vi "3d_display3.vi"() -> ()   [LabVIEW 2009]
doc: "This example demonstrates some fundamental concepts for the 3D picture control. Concepts covered include:\n\n-Object creation\n-Texturing\n-Object movement\n-Object hierarchy"
uses:
  <vilib>/Utility/miscctls.llb/LVRectTypeDef.ctl
  <vilib>/picture/3D Picture Control/NI_3D Picture Control.lvlib
  <vilib>/Analysis/NI_AALBase.lvlib
panel:
  out "xadd":dbl
  out "zadd":dbl
  out "raw pitot":dbl
  in  "Calibrate pitot":bool
  in  "voltage offset":dbl=2.5
  in  "velocity scale":dbl=10000.0
  in  "Set Start Time (s)":dbl
  in  "X":dbl
  in  "Z":dbl
  in  "Calibrate Z":bool
  in  "Calibrate Y":bool
  in  "Calibrate X":bool
  out "angle 2":dbl
  out "angle 1":dbl
  out "X mean acceleration":dbl format="%0.4f"
  out "Y mean acceleration":dbl format="%0.4f"
  out "X mean volts":dbl format="%0.4f"
  out "Y mean volts":dbl format="%0.4f"
  out "Z mean acceleration":dbl format="%0.4f"
  out "Z mean volts":dbl format="%0.4f"
  in  "z gain":dbl=5.0
  in  "z offset":dbl=1.25
  in  "y gain":dbl=5.0
  in  "y offset":dbl=1.25
  in  "x gain":dbl=5.0
  in  "x offset":dbl=1.25
  in  "Render Dest":enum16{"Scene Window", "Scene Display"}(ring)=enum."Scene Display"
  in  "Camera Controller":enum16{"None", "Spherical", "Flying"}(ring)=enum."Spherical"
  out "Scene Display":refnum<vi>(3d-picture)
  in  "stop":bool
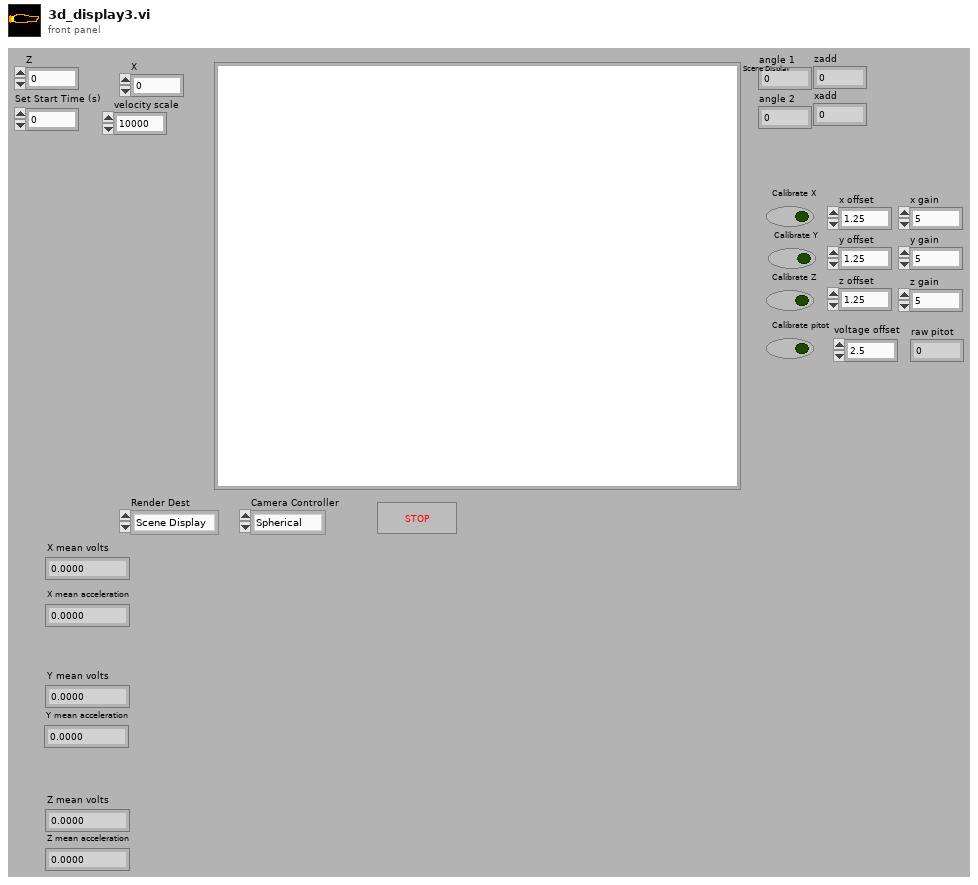
[diagram p1: front panel]
types:
  T1 = typedef "LVRectTypeDef.ctl" = cluster{"Left":i16, "Top":i16, "Right":i16, "Bottom":i16}
  T2 = enum16{"Open", "Minimized", "Maximized", "Hidden"}
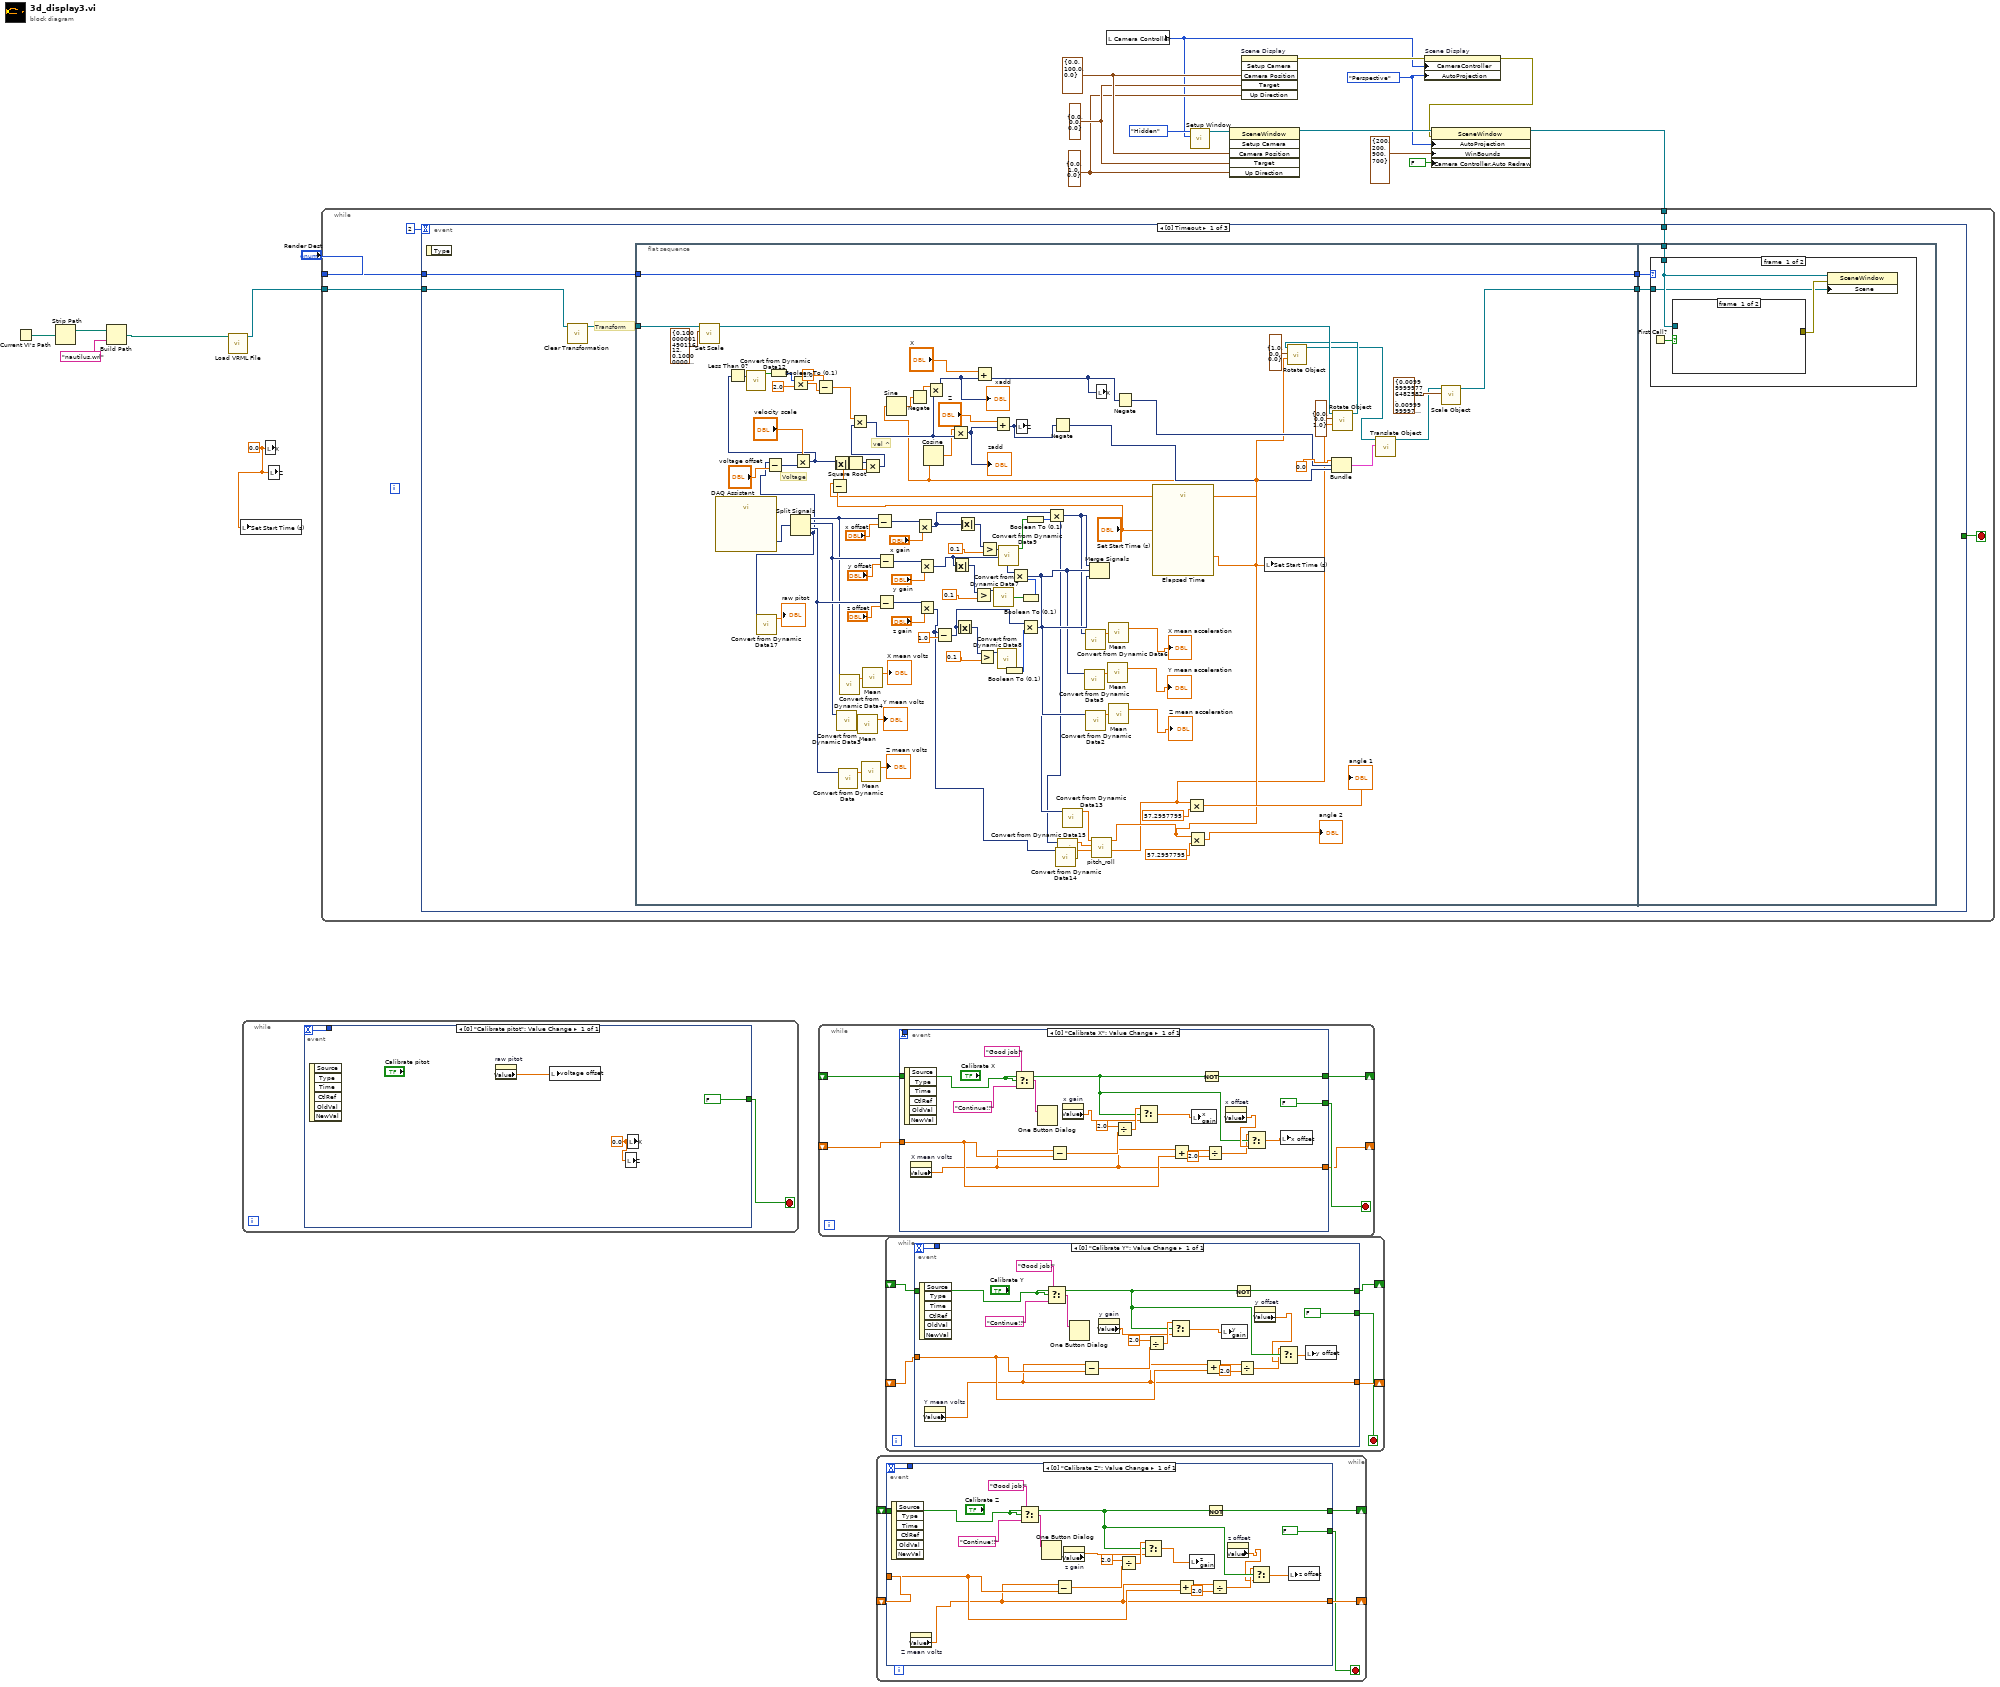
[diagram p0: block diagram]
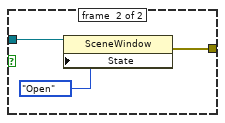
[diagram p2: hidden frame]
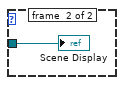
[diagram p3: hidden frame]
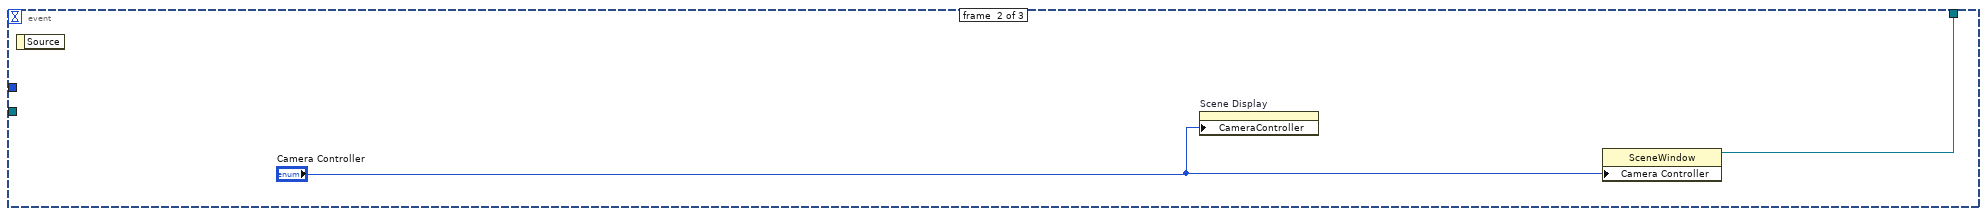
[diagram p4: hidden frame]
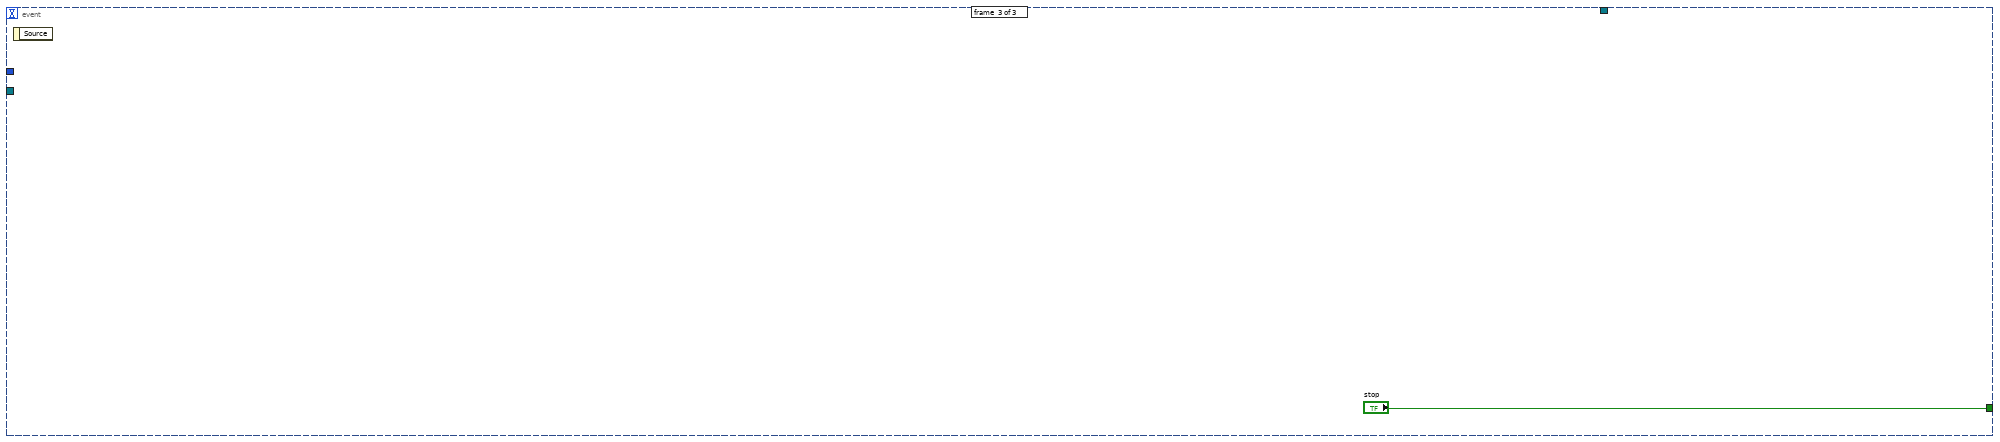
[diagram p5: hidden frame]
diagram:
  w1 = 0.0 ("X")
  w13 = enum16{"None", "Perspective", "Orthographic"}."Perspective" ("Auto Projection Mode")
  w16 = cluster{"X":sgl, "Y":sgl, "Z":sgl} {"X"=0.0, "Y"=1.0, "Z"=0.0} ("Up Direction")
  w17 = cluster{"X":sgl, "Y":sgl, "Z":sgl} {"X"=0.0, "Y"=0.0, "Z"=0.0} ("Target")
  w18 = cluster{"X":sgl, "Y":sgl, "Z":sgl} {"X"=0.0, "Y"=100.0, "Z"=0.0} ("Camera Position")
  n1 = Current VI's Path() -> (path=w5:path)
  n2 = Strip Path(path=w5) -> (stripped path=w6:path)  [unwired: 1 out]
  n3 = Build Path(base path=w6, name or relative path="nautilus.wrl") -> (appended path=w3:path)
  n4 = call <vilib>:"Load VRML File.vi"("Path"=w3) -> ("Scene:Read Scene File"=w2:refnum<vi>)  [unwired: 9 in, 1 out]
  n5 = local write "Set Start Time (s)"(w1) -> ()
  n6 = while {
    stop <- w21 stop-if-true
    n7 = event shown="[0] \"Calibrate pitot\": Value Change" {
      selector: _ -> [_]
      dyn-events: _ -> [_]
      timeout: _ -> [w25]
      tunnel: [w25] -> _
      tunnel: [FALSE ("Run")] -> w21
      event [0] "Calibrate pitot": Value Change {
        w22 = 0.0 ("X")
        n8 = event-data() -> ()  [unwired: 1 in, 6 out]
        n9 = property on="raw pitot" class="DigNum (strict)"() -> ("Value"=w23:dbl)  [unwired: 2 in, 2 out]
        n10 = local write "voltage offset"(w23) -> ()
        n11 = local write "Z"(w22) -> ()
        n12 = local write "X"(w22) -> ()
      }
    }
  }
  n13 = local write "X"(w1) -> ()
  n14 = local write "Z"(w1) -> ()
  n15 = while {
    shift-right: [w28] -> _
    shift-left: _ -> [w29]
    shift-right: [w27] -> _
    shift-left: _ -> [w26]
    stop <- w30 stop-if-true
    n16 = event shown="[0] \"Calibrate X\": Value Change" {
      selector: _ -> [_]
      dyn-events: _ -> [_]
      timeout: _ -> [w49]
      tunnel: [w49] -> _
      tunnel: [FALSE ("Run")] -> w30
      tunnel: w29 -> [w36]
      tunnel: [w44] -> w28
      tunnel: [w31] -> w27
      tunnel: w26 -> [w35]
      event [0] "Calibrate X": Value Change {
        n17 = event-data() -> ()  [unwired: 1 in, 6 out]
        n18 = property on="X mean volts" class="DigNum (strict)"() -> ("Value"=w31:dbl)  [unwired: 2 in, 2 out]
        n19 = Select(t="Good job!" ("message"), s=w36, f="Continue!!" ("message")) -> (s? t:f=w48:string)
        n20 = One Button Dialog(message=w48) -> ()  [unwired: 1 in, 1 out]
        n21 = Subtract(x=w31, y=w35) -> (x-y=w42:dbl)
        n22 = property on="x gain" class="DigNum (strict)"() -> ("Value"=w40:dbl)  [unwired: 2 in, 2 out]
        n23 = Divide(x=2.0, y=w42) -> (x/y=w41:dbl)
        n24 = Select(t=w41, s=w36, f=w40) -> (s? t:f=w39:dbl)
        n25 = Add(x=w31, y=w35) -> (x+y=w33:dbl)
        n26 = local write "x gain"(w39) -> ()
        n27 = Not(x=w36) -> (.not. x?=w44:bool)
        n28 = Divide(x=w33, y=2.0) -> (x/y=w32:dbl)
        n29 = property on="x offset" class="DigNum (strict)"() -> ("Value"=w37:dbl)  [unwired: 2 in, 2 out]
        n30 = Select(t=w32, s=w36, f=w37) -> (s? t:f=w38:dbl)
        n31 = local write "x offset"(w38) -> ()
      }
    }
  }
  n32 = while {
    shift-right: [w52] -> _
    shift-left: _ -> [w51]
    shift-right: [w54] -> _
    shift-left: _ -> [w53]
    stop <- w50 stop-if-true
    n33 = event shown="[0] \"Calibrate Z\": Value Change" {
      selector: _ -> [_]
      dyn-events: _ -> [_]
      timeout: _ -> [w73]
      tunnel: [w73] -> _
      tunnel: w53 -> [w65]
      tunnel: [w69] -> w54
      tunnel: [w55] -> w52
      tunnel: w51 -> [w64]
      tunnel: [FALSE ("Run")] -> w50
      event [0] "Calibrate Z": Value Change {
        n34 = event-data() -> ()  [unwired: 1 in, 6 out]
        n35 = property on="Z mean volts" class="DigNum (strict)"() -> ("Value"=w55:dbl)  [unwired: 2 in, 2 out]
        n36 = Select(t="Good job!" ("message"), s=w65, f="Continue!!" ("message")) -> (s? t:f=w72:string)
        n37 = One Button Dialog(message=w72) -> ()  [unwired: 1 in, 1 out]
        n38 = Subtract(x=w55, y=w64) -> (x-y=w67:dbl)
        n39 = property on="z gain" class="DigNum (strict)"() -> ("Value"=w59:dbl)  [unwired: 2 in, 2 out]
        n40 = Divide(x=2.0, y=w67) -> (x/y=w66:dbl)
        n41 = Select(t=w66, s=w65, f=w59) -> (s? t:f=w57:dbl)
        n42 = Add(x=w55, y=w64) -> (x+y=w62:dbl)
        n43 = local write "z gain"(w57) -> ()
        n44 = Not(x=w65) -> (.not. x?=w69:bool)
        n45 = Divide(x=w62, y=2.0) -> (x/y=w61:dbl)
        n46 = property on="z offset" class="DigNum (strict)"() -> ("Value"=w58:dbl)  [unwired: 2 in, 2 out]
        n47 = Select(t=w61, s=w65, f=w58) -> (s? t:f=w60:dbl)
        n48 = local write "z offset"(w60) -> ()
      }
    }
  }
  n49 = while {
    shift-right: [w78] -> _
    shift-left: _ -> [w77]
    shift-right: [w75] -> _
    shift-left: _ -> [w76]
    stop <- w74 stop-if-true
    n50 = event shown="[0] \"Calibrate Y\": Value Change" {
      selector: _ -> [_]
      dyn-events: _ -> [_]
      timeout: _ -> [w97]
      tunnel: [w97] -> _
      tunnel: w77 -> [w89]
      tunnel: [w93] -> w78
      tunnel: [w79] -> w75
      tunnel: w76 -> [w88]
      tunnel: [FALSE ("Run")] -> w74
      event [0] "Calibrate Y": Value Change {
        n51 = event-data() -> ()  [unwired: 1 in, 6 out]
        n52 = property on="Y mean volts" class="DigNum (strict)"() -> ("Value"=w79:dbl)  [unwired: 2 in, 2 out]
        n53 = Select(t="Good job!" ("message"), s=w89, f="Continue!!" ("message")) -> (s? t:f=w96:string)
        n54 = One Button Dialog(message=w96) -> ()  [unwired: 1 in, 1 out]
        n55 = Subtract(x=w79, y=w88) -> (x-y=w91:dbl)
        n56 = property on="y gain" class="DigNum (strict)"() -> ("Value"=w84:dbl)  [unwired: 2 in, 2 out]
        n57 = Divide(x=2.0, y=w91) -> (x/y=w90:dbl)
        n58 = Select(t=w90, s=w89, f=w84) -> (s? t:f=w83:dbl)
        n59 = Add(x=w79, y=w88) -> (x+y=w86:dbl)
        n60 = local write "y gain"(w83) -> ()
        n61 = Not(x=w89) -> (.not. x?=w93:bool)
        n62 = Divide(x=w86, y=2.0) -> (x/y=w85:dbl)
        n63 = property on="y offset" class="DigNum (strict)"() -> ("Value"=w82:dbl)  [unwired: 2 in, 2 out]
        n64 = Select(t=w85, s=w89, f=w82) -> (s? t:f=w81:dbl)
        n65 = local write "y offset"(w81) -> ()
      }
    }
  }
  n66 = local read "Camera Controller"() -> (w10:enum16{"None", "Spherical", "Flying"})
  n67 = call <vilib>:"Setup Window.vi"("Camera Controller"=w10, "Window State"=T2."Hidden") -> ("New Window Refnum"=w12:refnum<vi>)  [unwired: 1 in, 8 out]
  n68 = invoke class="SceneWindow" method="Setup Camera"(reference=w12, "Camera Position"=w18, "Target"=w17, "Up Direction"=w16) -> (reference out=w20:refnum<vi>)  [unwired: 2 in, 5 out]
  n69 = invoke on="Scene Display" class="SceneGraphDisp (strict)" method="Setup Camera"("Camera Position"=w18, "Target"=w17, "Up Direction"=w16) -> (error out=w15:errorcluster)  [unwired: 3 in, 5 out]
  n70 = property on="Scene Display" class="SceneGraphDisp (strict)"(error in=w15, "CameraController"=w10, "AutoProjection"=w13) -> (error out=w14:errorcluster)  [unwired: 1 in, 1 out]
  n71 = property class="SceneWindow"(reference=w20, error in=w14, "AutoProjection"=w13, "WinBounds"=T1 {"Left"=200, "Top"=200, "Right"=900, "Bottom"=700} ("Window Bounds"), "Camera Controller.Auto Redraw"=FALSE ("Camera Controller:Auto Redraw")) -> (reference out=w8:refnum<vi>)  [unwired: 1 out]
  n72 = while {
    tunnel: w8 -> [w102]
    tunnel: w2 -> [w101]
    tunnel: "Render Dest" -> [w98]
    stop <- w99 stop-if-true
    n73 = event shown="[0] Timeout" {
      selector: _ -> [_ _ _]
      dyn-events: _ -> [_ _ _]
      timeout: 2 -> [_ _ _]
      tunnel: w102 -> [w108 w222 _]
      tunnel: w101 -> [w104 _ _]
      tunnel: [_ _ "stop"] -> w99
      tunnel: w98 -> [w105 _ _]
      event #0 {
        # "Transform"
        n74 = event-data() -> ()  [unwired: 2 out]
        n75 = call <vilib>:"Clear Transformation.vi"("Object Refnum In"=w104) -> ("Object Refnum Out"=w107:refnum<vi>)  [unwired: 1 in, 9 out]
        n76 = flat-sequence {
          tunnel: w107 -> [w137]
          tunnel: [w209] -> w106
          tunnel: w105 -> [w209]
          tunnel: [w206] -> w103
          tunnel: w108 -> [w212]
          tunnel: w106 -> [w211]
          tunnel: w103 -> [w210]
          frame #0 {
            # "vel ^"
            # "Voltage"
            n77 = call <vilib>:"Set Scale.vi"("Scale"=cluster{"X":sgl, "Y":sgl, "Z":sgl} {"X"=0.1, "Y"=0.1, "Z"=0.1}, "Scene Object"=w137) -> ("Scaled Object"=w125:refnum<vi>)  [unwired: 8 in, 1 out]
            n78 = call "DAQ Assistant"() -> ("data"=w158:dynamicdata)  [unwired: 17 in, 2 out]
            n79 = Split Signals(w158) -> (w189:dynamicdata, w191:dynamicdata, w194:dynamicdata, w121:dynamicdata)  [unwired: 4 in]
            n80 = call "Convert from Dynamic Data17"("Dynamic Data Type"=w121) -> ("Scalar"=→"raw pitot":dbl)  [unwired: 3 in]
            n81 = Subtract(x=w121, y="voltage offset") -> (x-y=w156:dynamicdata)
            n82 = Multiply(x="velocity scale", y=w156) -> (x*y=w115:dynamicdata)
            n83 = Less Than 0?(x=w115) -> (x < 0?=w114:dynamicdata)
            n84 = call "Convert from Dynamic Data12"("Dynamic Data Type"=w114) -> ("Scalar"=w147:bool)  [unwired: 3 in]
            n85 = Boolean To (0,1)(Boolean=w147) -> (0, 1=w145:i16)
            n86 = Multiply(x=w145, y=2.0) -> (x*y=w143:dbl)
            n87 = Subtract(x=1.0 ("y"), y=w143) -> (x-y=w140:dbl)
            n88 = Absolute Value(x=w115) -> (abs(x)=w142:dynamicdata)
            n89 = call "Convert from Dynamic Data3"("Dynamic Data Type"=w191) -> ("Array"=w190:dbl[])  [unwired: 3 in]
            n90 = call "Convert from Dynamic Data"("Dynamic Data Type"=w194) -> ("Array"=w196:dbl[])  [unwired: 3 in]
            n91 = call "Convert from Dynamic Data4"("Dynamic Data Type"=w189) -> ("Array"=w188:dbl[])  [unwired: 3 in]
            n92 = Square Root(x=w142) -> (sqrt(x)=w141:dynamicdata)
            n93 = call <vilib>:"Mean.vi"("X"=w190) -> ("mean"=→"Y mean volts":dbl)  [unwired: 1 out]
            n94 = call <vilib>:"Mean.vi"("X"=w196) -> ("mean"=→"Z mean volts":dbl)  [unwired: 1 out]
            n95 = call <vilib>:"Mean.vi"("X"=w188) -> ("mean"=→"X mean volts":dbl)  [unwired: 1 out]
            n96 = Subtract(x=w189, y="x offset") -> (x-y=w205:dynamicdata)
            n97 = Subtract(x=w191, y="y offset") -> (x-y=w201:dynamicdata)
            n98 = Subtract(x=w194, y="z offset") -> (x-y=w183:dynamicdata)
            n99 = Multiply(x=w205, y="x gain") -> (x*y=w164:dynamicdata)
            n100 = Multiply(x=w201, y="y gain") -> (x*y=w182:dynamicdata)
            n101 = Multiply(x=w183, y="z gain") -> (x*y=w126:dynamicdata)
            n102 = Subtract(x=w126, y=1.0) -> (x-y=w170:dynamicdata)
            n103 = Absolute Value(x=w182) -> (abs(x)=w181:dynamicdata)
            n104 = Absolute Value(x=w170) -> (abs(x)=w176:dynamicdata)
            n105 = Absolute Value(x=w164) -> (abs(x)=w169:dynamicdata)
            n106 = Greater?(x=w181, y=0.1) -> (0:w178:dynamicdata)
            n107 = Greater?(x=w176, y=0.1) -> (0:w174:dynamicdata)
            n108 = Greater?(x=w169, y=0.1) -> (0:w166:dynamicdata)
            n109 = call "Convert from Dynamic Data7"("Dynamic Data Type"=w178) -> ("Scalar"=w177:bool)  [unwired: 3 in]
            n110 = call "Convert from Dynamic Data8"("Dynamic Data Type"=w174) -> ("Scalar"=w173:bool)  [unwired: 3 in]
            n111 = call "Convert from Dynamic Data9"("Dynamic Data Type"=w166) -> ("Scalar"=w165:bool)  [unwired: 3 in]
            n112 = Boolean To (0,1)(Boolean=w173) -> (0, 1=w172:i16)
            n113 = Boolean To (0,1)(Boolean=w177) -> (0, 1=w179:i16)
            n114 = Multiply(x=w182, y=w179) -> (x*y=w128:dynamicdata)
            n115 = Multiply(x=w170, y=w172) -> (x*y=w153:dynamicdata)
            n116 = Boolean To (0,1)(Boolean=w165) -> (0, 1=w167:i16)
            n117 = Multiply(x=w164, y=w167) -> (x*y=w127:dynamicdata)
            n118 = call "Convert from Dynamic Data14"("Dynamic Data Type"=w126) -> ("Scalar"=w112:dbl)  [unwired: 3 in]
            n119 = call "Convert from Dynamic Data15"("Dynamic Data Type"=w127) -> ("Scalar"=w111:dbl)  [unwired: 3 in]
            n120 = call "Convert from Dynamic Data13"("Dynamic Data Type"=w128) -> ("Scalar"=w113:dbl)  [unwired: 3 in]
            n121 = call "Convert from Dynamic Data5"("Dynamic Data Type"=w128) -> ("Array"=w185:dbl[])  [unwired: 3 in]
            n122 = call "Convert from Dynamic Data6"("Dynamic Data Type"=w127) -> ("Array"=w184:dbl[])  [unwired: 3 in]
            n123 = call "Convert from Dynamic Data2"("Dynamic Data Type"=w153) -> ("Array"=w195:dbl[])  [unwired: 3 in]
            n124 = Merge Signals(w127, w128, w153) -> ()  [unwired: 1 out]
            n125 = call "pitch_roll.vi"("Az"=w112, "Ay"=w111, "Ax"=w113) -> ("Pitch"=w109:dbl, "Roll"=w110:dbl)  [unwired: 7 in]
            n126 = Sine(x=w110) -> (sin(x)=w116:dbl)
            n127 = Negate(x=w116) -> (-x=w117:dbl)
            n128 = Cosine(x=w110) -> (cos(x)=w135:dbl)
            n129 = call <vilib>:"Mean.vi"("X"=w185) -> ("mean"=→"Y mean acceleration":dbl)  [unwired: 1 out]
            n130 = call <vilib>:"Mean.vi"("X"=w184) -> ("mean"=→"X mean acceleration":dbl)  [unwired: 1 out]
            n131 = call <vilib>:"Mean.vi"("X"=w195) -> ("mean"=→"Z mean acceleration":dbl)  [unwired: 1 out]
            n132 = call "Elapsed Time"("Set Start Time (s)"="Set Start Time (s)") -> ("Elapsed Time (s)"=w119:dbl)  [unwired: 11 in, 7 out]
            n133 = Subtract(x=w119, y="Set Start Time (s)") -> (x-y=w148:dbl)
            n134 = Multiply(x=w141, y=w148) -> (x*y=w139:dynamicdata)
            n135 = Multiply(x=w140, y=w139) -> (x*y=w138:dynamicdata)
            n136 = Multiply(x=w117, y=w138) -> (x*y=w118:dynamicdata)
            "xadd" <- w118
            n137 = Multiply(x=w135, y=w138) -> (x*y=w152:dynamicdata)
            "zadd" <- w152
            n138 = Add(x="X", y=w118) -> (x+y=w130:dynamicdata)
            n139 = Add(x="Z", y=w152) -> (x+y=w132:dynamicdata)
            n140 = local write "Z"(w132) -> ()
            n141 = Negate(x=w132) -> (-x=w131:dynamicdata)
            n142 = local write "X"(w130) -> ()
            n143 = Negate(x=w130) -> (-x=w129:dynamicdata)
            n144 = Multiply(x=w109, y=57.2957795) -> (x*y=→"angle 1":dbl)
            n145 = Multiply(x=w110, y=57.2957795) -> (x*y=→"angle 2":dbl)
            n146 = local write "Set Start Time (s)"(w119) -> ()
            n147 = Bundle("element"=0.0, w129, w131) -> (w150:cluster{"element":dbl, dynamicdata, dynamicdata})  [unwired: 1 in]
            n148 = call <vilib>:"Rotate Object.vi"("Angle"=w109, "Axis"=cluster{"X":sgl, "Y":sgl, "Z":sgl} {"X"=0.0, "Y"=0.0, "Z"=1.0}, "Scene.Object In"=w125) -> ("Scene.Object Out"=w124:refnum<vi>)  [unwired: 7 in, 1 out]
            n149 = call <vilib>:"Rotate Object.vi"("Angle"=w110, "Axis"=cluster{"X":sgl, "Y":sgl, "Z":sgl} {"X"=1.0, "Y"=0.0, "Z"=0.0}, "Scene.Object In"=w124) -> ("Scene.Object Out"=w123:refnum<vi>)  [unwired: 7 in, 1 out]
            n150 = call <vilib>:"Translate Object.vi"("Translation"=w150, "Scene.Object In"=w123) -> ("Scene.Object Out"=w151:refnum<vi>)  [unwired: 8 in, 1 out]
            n151 = call <vilib>:"Scale Object.vi"("Scale"=cluster{"X":sgl, "Y":sgl, "Z":sgl} {"X"=0.01, "Y"=0.01, "Z"=0.01}, "Scene.Object In"=w151) -> ("Scene.Object Out"=w206:refnum<vi>)  [unwired: 8 in, 1 out]
          }
          frame #1 {
            n152 = case shown="\"Scene Window\", Default" w211 {
              tunnel: w212 -> [w216 _]
              tunnel: w210 -> [w213 w220]
              frame #0 {
                n153 = First Call?() -> (First Call?: T/F=w214:bool)
                n154 = case shown="True" w214 {
                  tunnel: w216 -> [_ w219]
                  tunnel: [_ w218] -> w215
                  frame #0 {
                  }
                  frame #1 {
                    n155 = property class="SceneWindow"(reference=w219, "State"=T2."Open" ("Window State")) -> (error out=w218:errorcluster)  [unwired: 1 in, 1 out]
                  }
                }
                n156 = property class="SceneWindow"(reference=w216, error in=w215, "Scene"=w213) -> ()  [unwired: 2 out]
              }
              frame #1 {
                "Scene Display" <- w220
              }
            }
          }
        }
      }
      event #1 {
        n157 = event-data() -> ()  [unwired: 2 out]
        n158 = property on="Scene Display" class="SceneGraphDisp (strict)"("CameraController"="Camera Controller") -> ()  [unwired: 2 in, 2 out]
        n159 = property class="SceneWindow"(reference=w222, "Camera Controller"="Camera Controller") -> ()  [unwired: 1 in, 2 out]
      }
      event #2 {
        n160 = event-data() -> ()  [unwired: 2 out]
      }
    }
  }
